vi "Infiray_project (1).vi"() -> ()   [LabVIEW 2021]
uses:
  <vilib>/userDefined/High Color/IMAQdx.ctl
  <vilib>/vision/driver/IMAQdx.llb/IMAQdx Attribute Type.ctl
  <vilib>/vision/driver/NI_Vision_Acquisition_Software.lvlib
  <resource>/objmgr/imaqdx.rc
  <vilib>/vision/NI_Vision_Development_Module.lvlib
panel:
  out "Attribute Information Array":T2(array[cluster])
  out "Área":dbl
  out "Alto":dbl
  out "Ancho":dbl
  out "Tmax_box (ºC)":dbl
  out "Gráfica Tmax_box":dbl(graph)
  out "Thermometer":dbl(slide) scale=0.0..200.0
  out "Last Mouse Position":cluster{"X":i32, "Y":i32}
  out "Temperature View":T3(plugin-control)
  out "Temperatura (ºC)":dbl
  in  "stop":bool
  in  "Number of Buffers":u32=5
  in  "Session In":T4
  # "PROPIEDADES RECTÁNGULO"
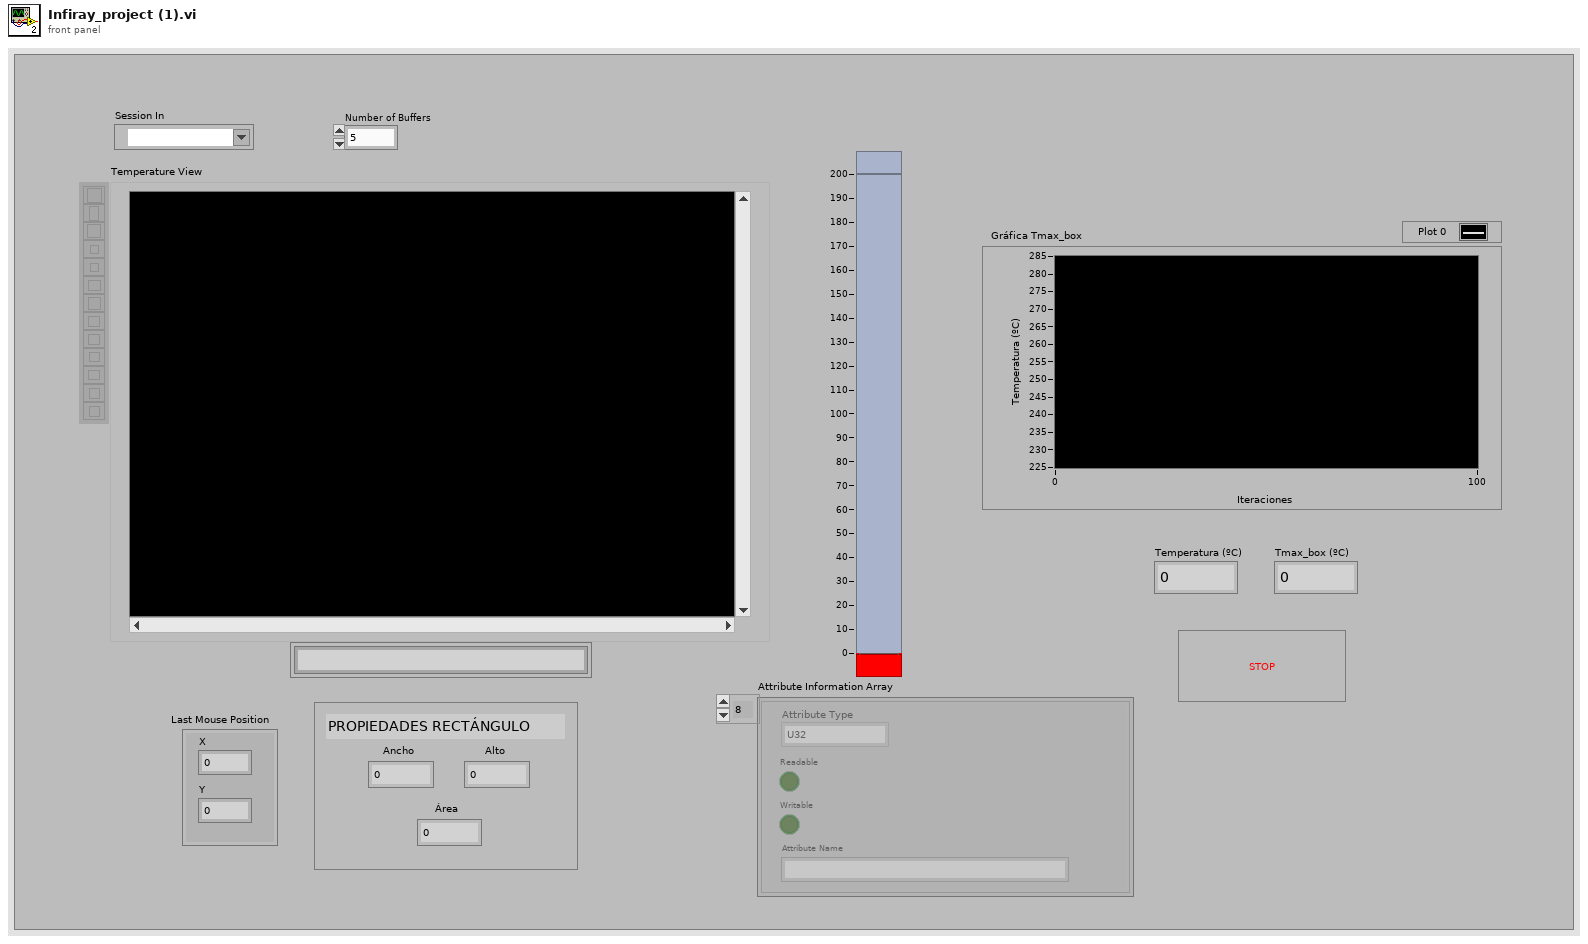
[diagram p1: front panel]
types:
  T1 = typedef "NI_Vision_Acquisition_Software.lvlib/IMAQdx Attribute Type.ctl" = enum32{"U32", "I64", "DBL", "String", "Enum", "Bool", "Command"}
  T2 = cluster{"Attribute Type":T1, "Readable":bool, "Writable":bool, "Attribute Name":string}[]
  T3 = typedef "IMAQ Image.ctl" = refnum<image>
  T4 = typedef "IMAQdx.ctl" = refnum<k21>
  T5 = typedef "Image Type" = u32
  T6 = cluster{"Global Rectangle":i32[], "Contours":cluster{"Contour Type":u32, "ROI Type":u32, "Points":i32[]}[]}
  T7 = typedef "IMAQ Rectangle" = cluster{"Left":i32, "Top":i32, "Right":i32, "Bottom":i32, "Rotation":dbl}
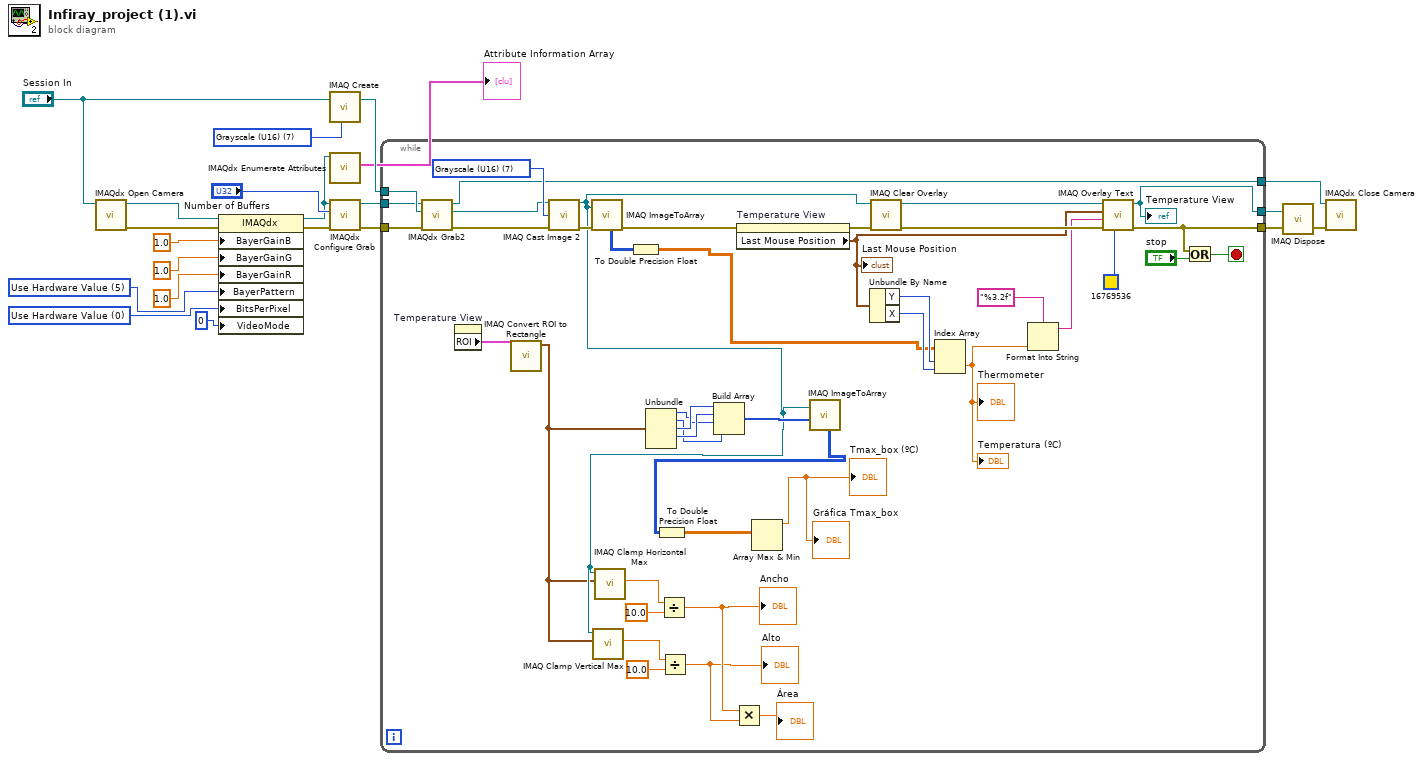
[diagram p0: block diagram]
diagram:
  w11 = u32 0 items=["Use Hardware Value"=0, "10-bit"=10, "12-bit"=12, "14-bit"=14, "16-bit"=16] ("BitsPerPixel")
  w12 = u32 5 items=["None", "GB", "GR", "BG", "RG", "Use Hardware Value"] ("BayerPattern")
  w16 = T5 7 items=["Grayscale (U8)", "Grayscale (I16)", "Grayscale (SGL)", "Complex (CSG)", "RGB (U32)", "HSL (U32)", "RGB (U64)", "Grayscale (U16)"] ("Image Type")
  n1 = call <vilib>:"IMAQdx Open Camera.vi"("Session In"="Session In") -> ("error out"=w8:errorcluster, "Session Out"=w9:T4)  [unwired: 9 in]
  n2 = property class="IMAQdx"(reference=w9, error in=w8, "BayerGainB"=1.0, "BayerGainG"=1.0, "BayerGainR"=1.0, "BayerPattern"=w12, "BitsPerPixel"=w11, "VideoMode"=u32 0) -> (reference out=w2:T4, error out=w7:errorcluster)
  n3 = call "IMAQ Create"("Image Name"="Session In", "Image Type"=w16) -> ("New Image"=w17:T3)  [unwired: 3 in, 1 out]
  n4 = call <vilib>:"IMAQdx Enumerate Attributes.vi"("Session In"=w2) -> ("Attribute Information Array"=→"Attribute Information Array":T2)  [unwired: 8 in, 2 out]
  n5 = call <vilib>:"IMAQdx Configure Grab.vi"("error in"=w7, "Number of Buffers"="Number of Buffers", "Session In"=w2) -> ("error out"=w19:errorcluster, "Session Out"=w20:T4)  [unwired: 7 in]
  n6 = while {
    tunnel: w17 -> [w64]
    tunnel: w20 -> [w41]
    tunnel: [w46] -> w6
    tunnel: w19 -> [w42]
    tunnel: [w51] -> w4
    tunnel: [w45] -> w5
    stop <- w62 stop-if-true
    w50 = T5 7 items=["Grayscale (U8)", "Grayscale (I16)", "Grayscale (SGL)", "Complex (CSG)", "RGB (U32)", "HSL (U32)", "RGB (U64)", "Grayscale (U16)"] ("Image Type")
    n7 = call <vilib>:"IMAQdx Grab2.vi"("error in"=w42, "Image In"=w64, "Session In"=w41) -> ("error out"=w61:errorcluster, "Image Out"=w49:T3, "Session Out"=w46:T4)  [unwired: 5 in, 1 out]
    n8 = property on="Temperature View" class="ImageControl"() -> ("ROI"=w39:T6)  [unwired: 2 in, 2 out]
    n9 = call "IMAQ Convert ROI to Rectangle"("ROI Descriptor"=w39) -> ("Rectangle"=w30:T7)  [unwired: 8 in, 1 out]
    n10 = call "IMAQ Cast Image 2"("Image Src"=w49, "Image Type"=w50, "error in (no error)"=w61) -> ("Image Dst Out"=w31:T3, "error out"=w52:errorcluster)  [unwired: 11 in]
    n11 = call "IMAQ ImageToArray"("error in (no error)"=w52, "Image"=w31) -> ("Image Pixels (U16)"=w44:u16[][], "error out"=w47:errorcluster)  [unwired: 2 in, 3 out]
    n12 = call "IMAQ Clamp Vertical Max"("Rectangle"=w30, "Image"=w31) -> ("Distance"=w27:sgl)  [unwired: 5 in, 4 out]
    n13 = call "IMAQ Clamp Horizontal Max"("Rectangle"=w30, "Image"=w31) -> ("Distance"=w26:sgl)  [unwired: 5 in, 4 out]
    n14 = To Double Precision Float(number=w44) -> (double precision float=w40:dbl[][])
    n15 = Unbundle(w30) -> ("Left"=w32:i32, "Top"=w33:i32, "Right"=w34:i32, "Bottom"=w35:i32)  [unwired: 1 out]
    n16 = Divide(x=w26, y=10.0) -> (x/y=w25:dbl)
    "Ancho" <- w25
    n17 = Divide(x=w27, y=10.0) -> (x/y=w24:dbl)
    "Alto" <- w24
    n18 = Build Array(w34, w35, w32, w33) -> (w38:i32[])
    n19 = Multiply(x=w25, y=w24) -> (x*y=→"Área":dbl)
    n20 = property on="Temperature View" class="ImageControl"(error in=w47) -> (error out=w48:errorcluster, "Last Mouse Position"=w55:cluster{"X":i32, "Y":i32})  [unwired: 1 in, 1 out]
    "Last Mouse Position" <- w55
    n21 = call "IMAQ ImageToArray"("Optional Rectangle"=w38, "Image"=w31) -> ("Image Pixels (U16)"=w22:u16[][])  [unwired: 2 in, 4 out]
    n22 = To Double Precision Float(number=w22) -> (double precision float=w37:dbl[][])
    n23 = Array Max & Min(array=w37) -> (max value=→"Tmax_box (ºC)" →"Gráfica Tmax_box":dbl)  [unwired: 3 out]
    n24 = Unbundle By Name(w55) -> ("Y"=w58:i32, "X"=w57:i32)
    n25 = call "IMAQ Clear Overlay"("error in (no error)"=w48, "Image"=w31) -> ("error out"=w59:errorcluster, "Image Out"=w60:T3)  [unwired: 8 in]
    n26 = Index Array(array=w40, index (row)=w58, index (col)=w57) -> (element=w43:dbl)
    "Temperatura (ºC)" <- w43
    "Thermometer" <- w43
    n27 = Format Into String(format string="%3.2f", w43) -> (resulting string=w56:string)  [unwired: 2 in, 1 out]
    n28 = call "IMAQ Overlay Text"("Text Color (black)"=u32 16769536, "error in (no error)"=w59, "String"=w56, "Origin"=w55, "Image"=w60) -> ("error out"=w51:errorcluster, "Image Out"=w45:T3)  [unwired: 5 in]
    "Temperature View" <- w45
    n29 = Or(x=w51, y="stop") -> (x .or. y?=w62:bool)
  }
  n30 = call "IMAQ Dispose"("Image"=w5, "error in (no error)"=w4) -> ("error out"=w3:errorcluster)  [unwired: 4 in]
  n31 = call <vilib>:"IMAQdx Close Camera.vi"("error in"=w3, "Session In"=w6) -> ()  [unwired: 9 in, 1 out]
